vi "Time FGV.vi"(10 "목표 시간":dbl, 11 "Time FGV 상태":enum16{"초기화", "카운팅"}(ring)) -> (2 "도달?":bool, 3 "현재 시간":dbl)   [LabVIEW 2020]
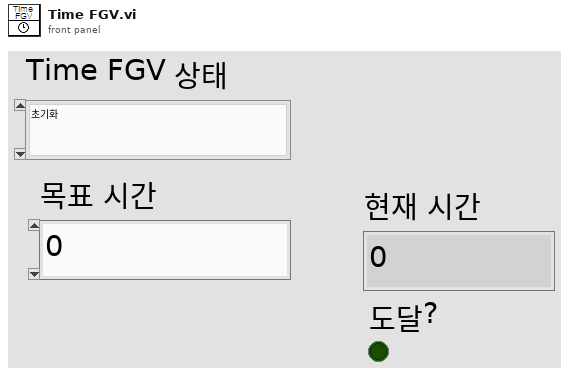
[diagram p1: front panel]
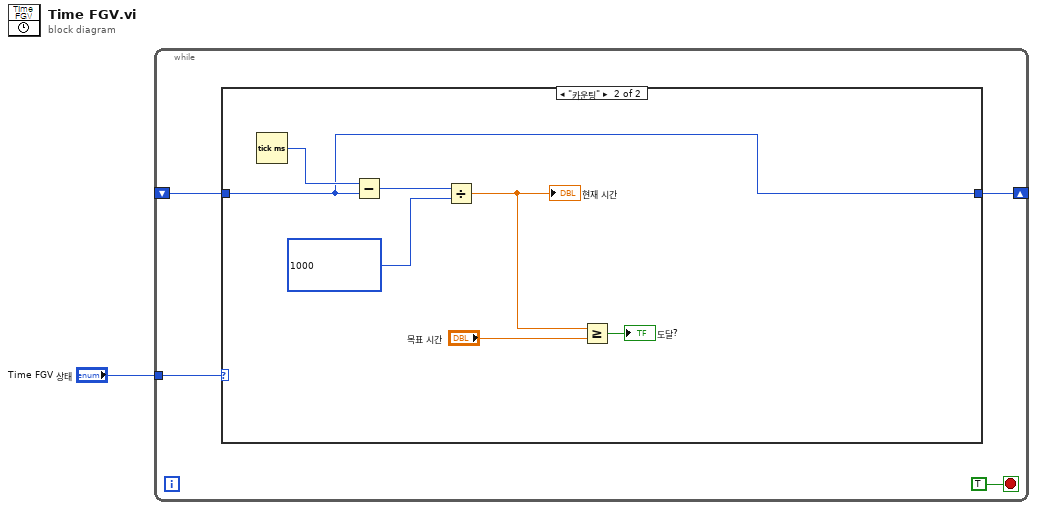
[diagram p0: block diagram]
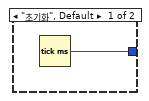
[diagram p2: hidden frame]
diagram:
  n1 = while {
    shift-right: [w3] -> _
    shift-left: _ -> [w2]
    tunnel: "Time FGV 상태" -> [w4]
    stop <- TRUE stop-if-true
    n2 = case shown="\"카운팅\"" w4 {
      tunnel: [w6 w7] -> w3
      tunnel: w2 -> [_ w7]
      frame "초기화", Default {
        n3 = Tick Count (ms)() -> (millisecond timer value=w6:u32)
      }
      frame "카운팅" {
        n4 = Tick Count (ms)() -> (millisecond timer value=w13:u32)
        n5 = Subtract(x=w13, y=w7) -> (x-y=w12:u32)
        n6 = Divide(x=w12, y=u32 1000) -> (x/y=w10:dbl)
        "현재 시간" <- w10
        n7 = Greater Or Equal?(x=w10, y="목표 시간") -> (x >= y?=→"도달?":bool)
      }
    }
  }
